vi "Test Save Snapshot.vi"() -> (0 "error out":errorcluster)   [LabVIEW 2020]
doc: "Test saving Snapshots with different settings."
uses:
  <vilib>/addons/_JKI Toolkits/Caraya/classes/Test/Test.lvclass
  src/Public API.lvlib
  src/Path Getter Mock/Path Getter Mock.lvclass
  src/Type Definitions/Snapshot Handling Options--cluster.ctl
  C:/Users/juanj/Documents/hasbun_wood_engineering/github/Debug-Snapshots-for-LabVIEW/src/Path Getter Mock/Path Getter Mock.lvclass
  C:/Users/juanj/Documents/hasbun_wood_engineering/github/Debug-Snapshots-for-LabVIEW/src/IPath Getter/IPath Getter.lvclass
  <vilib>/Utility/miscctls.llb/LVBreakpointStatusEnum.ctl
  src/Type Definitions/Class Name--enum.ctl
  src/Type Definitions/Breakpoint--cluster.ctl
  src/Type Definitions/Debug Snapshot--cluster.ctl
  src/Type Definitions/Debug Snapshot Array--cluster.ctl
  <vilib>/addons/_JKI Toolkits/Caraya/classes/Assert/Assert.lvclass
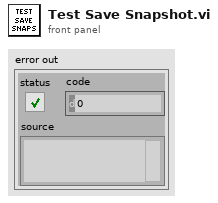
[diagram p1: front panel]
types:
  T1 = typedef "Debug Snapshot--cluster.ctl" = cluster{"VI Name":string, "Breakpoints":T2[], "Probes":i32[]}
  T2 = typedef "Breakpoint--cluster.ctl" = cluster{"UID":i32, "BP Status":T3, "Class Name":T4}
  T3 = typedef "LVBreakpointStatusEnum.ctl" = enum8{"Cleared Break", "Enabled Break", "Disabled Break"}
  T4 = typedef "Class Name--enum.ctl" = enum16{"Node", "Wire"}
  T5 = typedef "Snapshot Handling Options--cluster.ctl" = cluster{"Breakpoints":bool, "Probes":bool}
  T6 = typedef "Debug Snapshot Array--cluster.ctl" = cluster{"Debug Snapshots":T1[]}
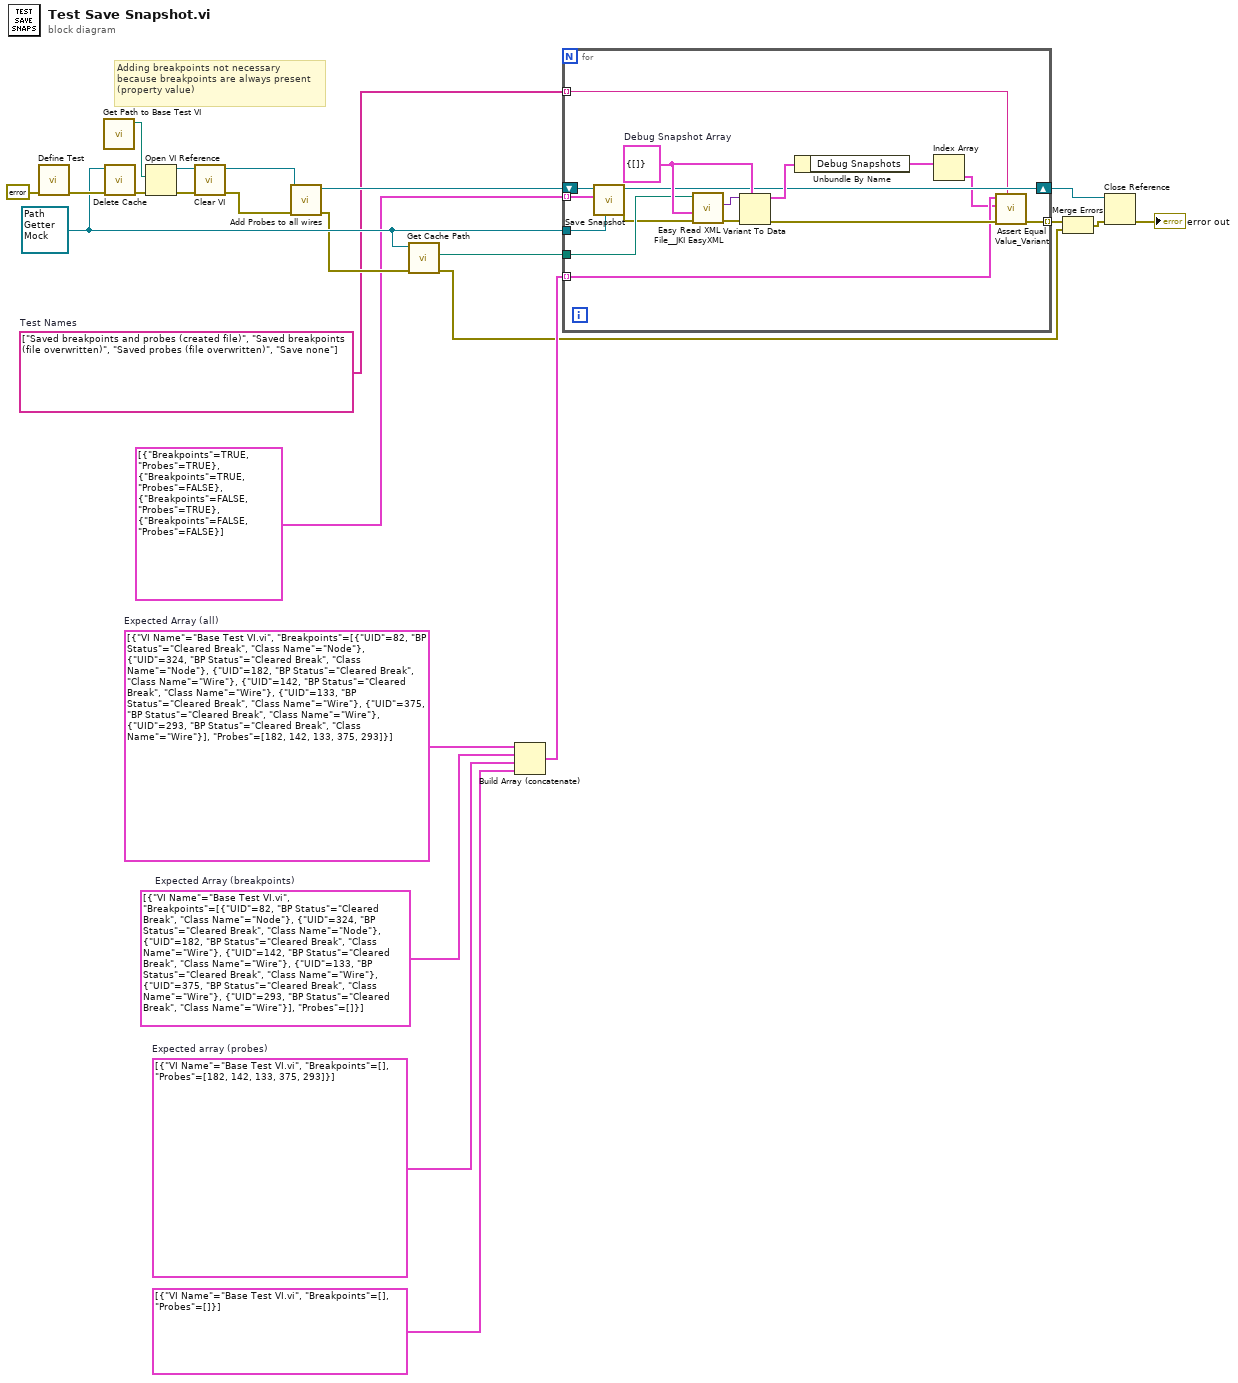
[diagram p0: block diagram]
diagram:
  w6 = T1[] [{"VI Name"="Base Test VI.vi", "Breakpoints"=[], "Probes"=[182, 142, 133, 375, 293]}]  # Expected array (probes)
  w13 = string[] ["Saved breakpoints and probes (created file)", "Saved breakpoints (file overwritten)", "Saved probes (file overwritten)", "Save none"]  # Test Names
  w7 = T1[] [{"VI Name"="Base Test VI.vi", "Breakpoints"=[{"UID"=82, "BP Status"=enum."Cleared Break", "Class Name"=enum."Node"}, {"UID"=324, "BP Status"=enum."Cleared Break", "Class Name"=enum."Node"}, {"UID"=182, "BP Status"=enum."Cleared Break", "Class Name"=enum."Wire"}, {"UID"=142, "BP Status"=enum."Cleared Break", "Class Name"=enum."Wire"}, {"UID"=133, "BP Status"=enum."Cleared Break", "Class Name"=enum."Wire"}, {"UID"=375, "BP Status"=enum."Cleared Break", "Class Name"=enum."Wire"}, {"UID"=293, "BP Status"=enum."Cleared Break", "Class Name"=enum."Wire"}], "Probes"=[]}]  # Expected Array (breakpoints)
  w12 = T1[] [{"VI Name"="Base Test VI.vi", "Breakpoints"=[{"UID"=82, "BP Status"=enum."Cleared Break", "Class Name"=enum."Node"}, {"UID"=324, "BP Status"=enum."Cleared Break", "Class Name"=enum."Node"}, {"UID"=182, "BP Status"=enum."Cleared Break", "Class Name"=enum."Wire"}, {"UID"=142, "BP Status"=enum."Cleared Break", "Class Name"=enum."Wire"}, {"UID"=133, "BP Status"=enum."Cleared Break", "Class Name"=enum."Wire"}, {"UID"=375, "BP Status"=enum."Cleared Break", "Class Name"=enum."Wire"}, {"UID"=293, "BP Status"=enum."Cleared Break", "Class Name"=enum."Wire"}], "Probes"=[182, 142, 133, 375, 293]}]  # Expected Array (all)
  w16 = refnum<class "Path Getter Mock.lvclass"> refnum ("Path Getter Mock.lvclass")
  # "Adding breakpoints not necessary\nbecause breakpoints are always present\n(property value)"
  n1 = call <vilib>:"Define Test.vi"("error in (no error)"=errorcluster {"status"=FALSE, "code"=0, "source"=""}) -> ("error out"=w21:errorcluster)  [unwired: 9 in, 1 out]
  n2 = call "Get Path to Base Test VI.vi"() -> ("Path"=w18:path)  [unwired: 11 in]
  n3 = call "Delete Cache.vi"("error in"=w21, "IPath Getter.lvclass"=w16) -> ("error out"=w23:errorcluster)  [unwired: 9 in]
  n4 = Open VI Reference(vi path=w18, error in (no error)=w23) -> (vi reference=w2:refnum<vi>, error out=w19:errorcluster)  [unwired: 4 in]
  n5 = call "Clear VI.vi"("error in"=w19, "VI Refnum In"=w2) -> ("error out"=w3:errorcluster, "VI Refnum Out"=w1:refnum<vi>)  [unwired: 8 in]
  n6 = call "Add Probes to all wires.vi"("error in"=w3, "VI Refnum In"=w1) -> ("error out"=w15:errorcluster, "VI Refnum Out"=w20:refnum<vi>)  [unwired: 8 in]
  n7 = call-dynamic "Get Cache Path.vi"("error in"=w15, "Path Getter Mock in"=w16) -> ("error out"=w4:errorcluster, "Path"=w17:path)  [unwired: 8 in]
  n8 = Build Array (concatenate)(w12, w7, w6, T1[] [{"VI Name"="Base Test VI.vi", "Breakpoints"=[], "Probes"=[]}] ("array")) -> (w11:T1[])
  n9 = for {
    tunnel: T5[] [{"Breakpoints"=TRUE, "Probes"=TRUE}, {"Breakpoints"=TRUE, "Probes"=FALSE}, {"Breakpoints"=FALSE, "Probes"=TRUE}, {"Breakpoints"=FALSE, "Probes"=FALSE}] ("Array") -> [w38] mode=indexing
    tunnel: w17 -> [w32]
    tunnel: w16 -> [w31]
    shift-right: [w33] -> w10
    shift-left: w20 -> [w39]
    tunnel: w13 -> [w29] mode=indexing
    tunnel: w11 -> [w28] mode=indexing
    tunnel: [w27] -> w9 mode=indexing
    w35 = T6 {"Debug Snapshots"=[]}  # Debug Snapshot Array
    n10 = call "Save Snapshot.vi"("IPath Getter in"=w31, "Debug Elements Options"=w38, "VI Reference in"=w39) -> ("error out"=w30:errorcluster, "VI Reference out"=w33:refnum<vi>)  [unwired: 7 in]
    n11 = call <vilib>:"Easy Read XML File__JKI EasyXML.vi"("error in (no error)"=w30, "LabVIEW Data (Type)"=w35, "XML File Path"=w32) -> ("error out"=w36:errorcluster, "LabVIEW Data"=w37:variant)  [unwired: 6 in, 1 out]
    n12 = Variant To Data(error in=w36, type=w35, Variant=w37) -> (data=w40:T6, error out=w34:errorcluster)
    n13 = Unbundle By Name(w40) -> ("Debug Snapshots"=w26:T1[])
    n14 = Index Array(array=w26) -> (element=w25:T1)  [unwired: 1 in]
    n15 = call <vilib>:"Assert Equal Value_Variant.vi"("Label"=w29, "error in (no error)"=w34, "Actual"=w25, "Expected"=w28) -> ("error out"=w27:errorcluster)  [unwired: 6 in, 1 out]
  }
  n16 = Merge Errors(w9, w4) -> (w8:errorcluster)
  n17 = Close Reference(reference=w10, error in (no error)=w8) -> (error out=→"error out":errorcluster)
